vi "Is part of the LabVIEW install folder.vi"(8 "error in (no error)":errorcluster, 11 "VI Reference":refnum<vi>) -> (0 "error out":errorcluster, 3 "Is part of LabVIEW install folder":bool)   [LabVIEW 2021]
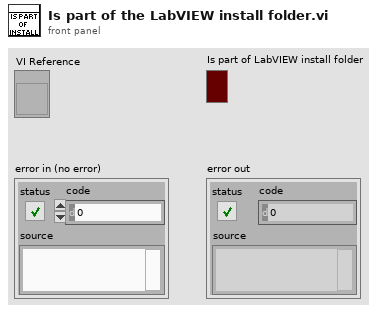
[diagram p1: front panel]
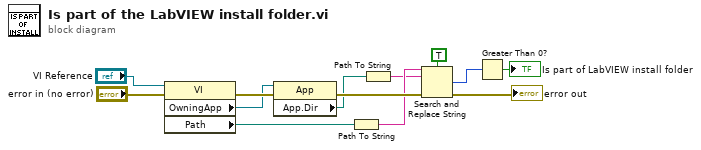
[diagram p0: block diagram]
diagram:
  n1 = property class="VI"(reference="VI Reference", error in="error in (no error)") -> (error out=w9:errorcluster, "OwningApp"=w8:refnum<vi>, "Path"=w4:path)  [unwired: 1 out]
  n2 = property class="App"(reference=w8, error in=w9) -> (error out=w6:errorcluster, "App.Dir"=w5:path)  [unwired: 1 out]
  n3 = Path To String(path=w4) -> (string=w3:string)
  n4 = Path To String(path=w5) -> (string=w2:string)
  n5 = Search and Replace String(case sensitive?=TRUE ("ignore case? (F)"), input string=w3, search string=w2, error in=w6) -> (number of replacements=w7:i32, error out=→"error out":errorcluster)  [unwired: 4 in, 2 out]
  n6 = Greater Than 0?(x=w7) -> (x > 0?=→"Is part of LabVIEW install folder":bool)
